vi "AlGaInPAs_Layer2.vi"(2 "Debug Mode":bool, 4 "State":enum16{"Edit", "Start", "Run", "End", "Idle"}(ring), 5 "Argument List In":string[](array[string])) -> (1 "Argument List Out":string[](array[string]))   [LabVIEW 2011]
panel:
  in  "AsH3 Flow":dbl
  in  "AsH3 run":bool
  in  "Al_run":bool
  in  "Al Flow":dbl
  in  "PH3 run":bool
  in  "In run":bool
  in  "Ga run":bool
  in  "PH3 Flow":dbl
  in  "In Flow":dbl
  in  "Ga Flow":dbl
  in  "Cancel":bool
  in  "OK":bool
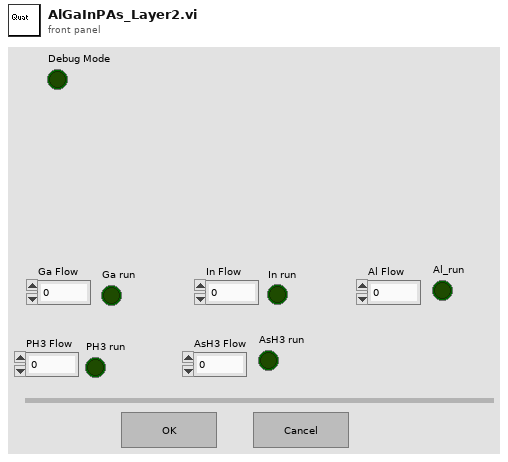
[diagram p1: front panel]
types:
  T1 = enum16{"Discrete", "Continuous", "Instantaneous"}
  T2 = enum32{"Invalid", "Default", "Floating", "Floating/Auto-Hide", "Modal"}
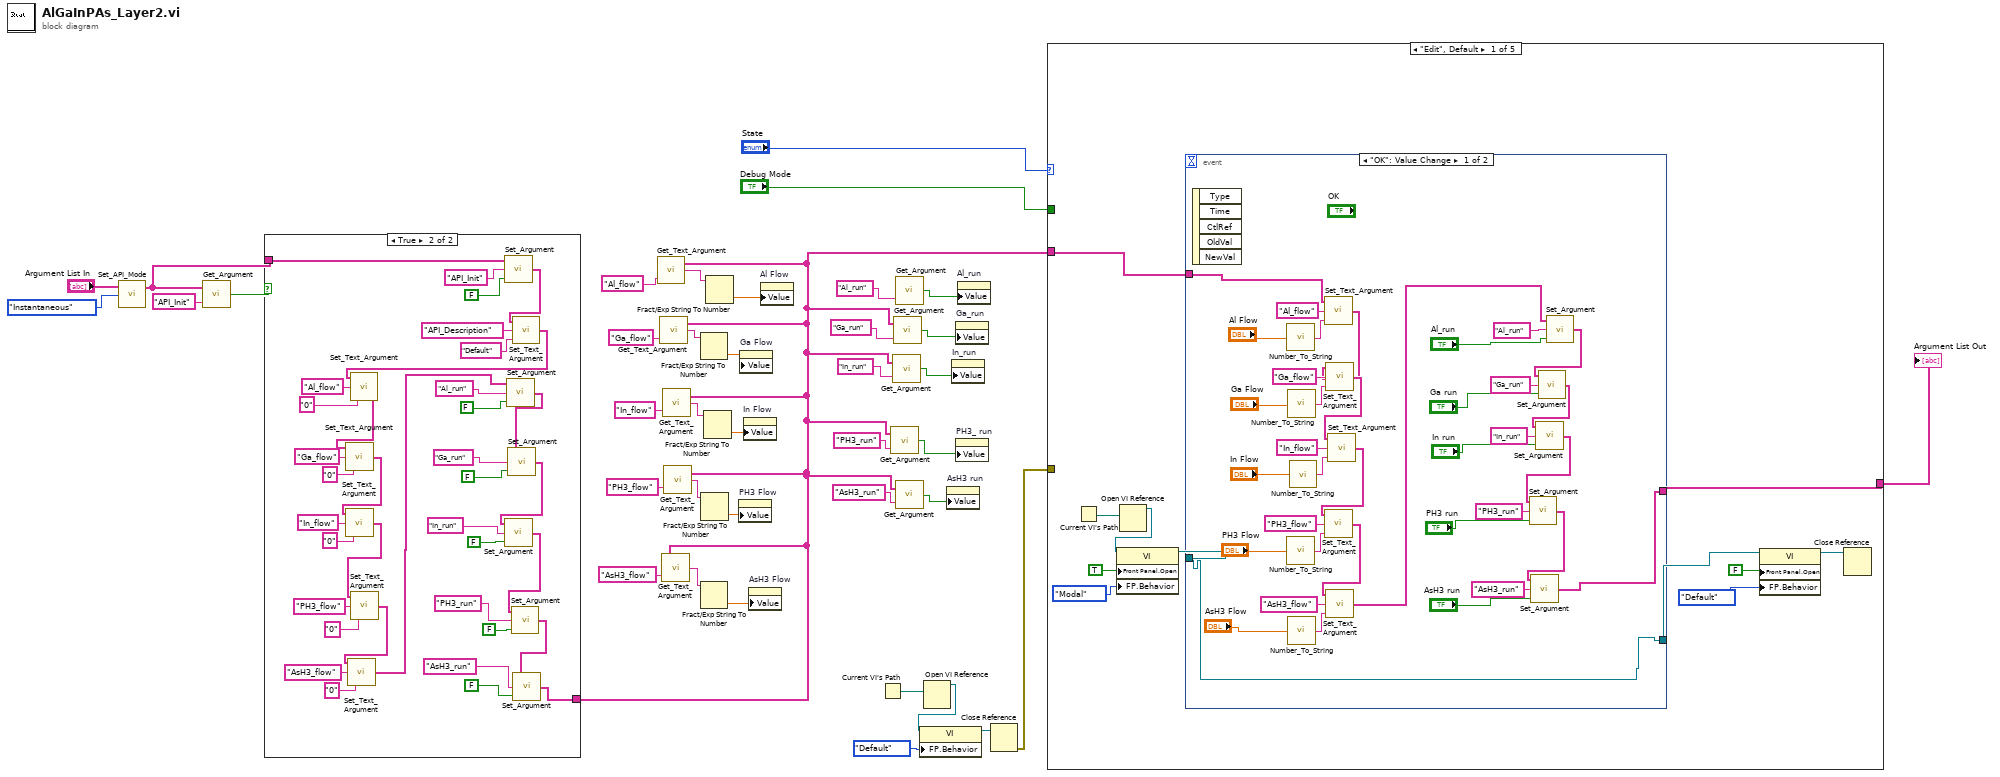
[diagram p0: block diagram]
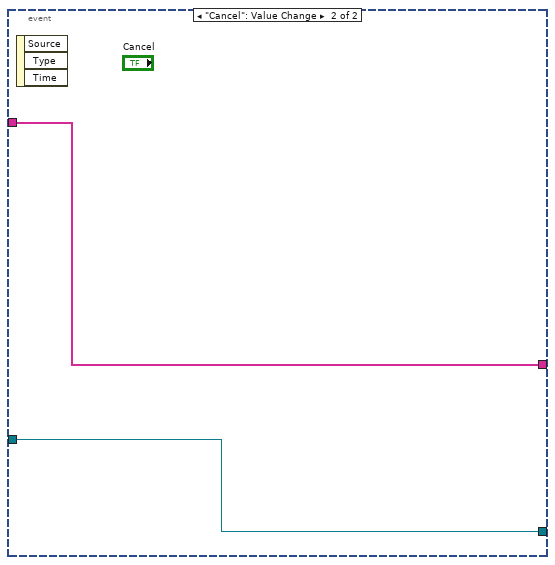
[diagram p3: hidden frame]
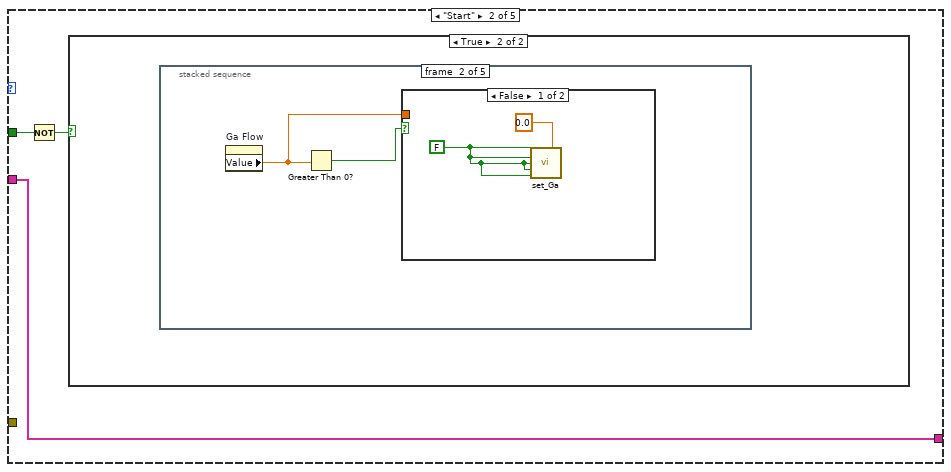
[diagram p4: hidden frame]
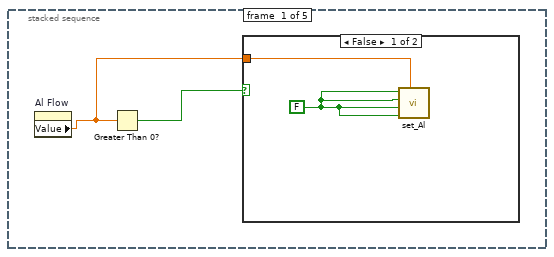
[diagram p6: hidden frame]
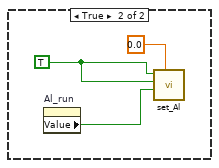
[diagram p7: hidden frame]
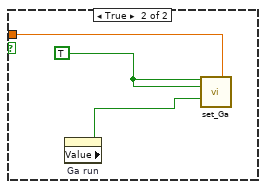
[diagram p8: hidden frame]
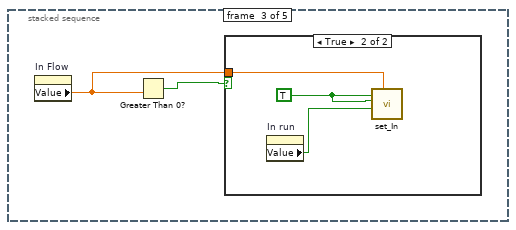
[diagram p9: hidden frame]
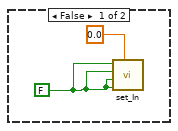
[diagram p10: hidden frame]
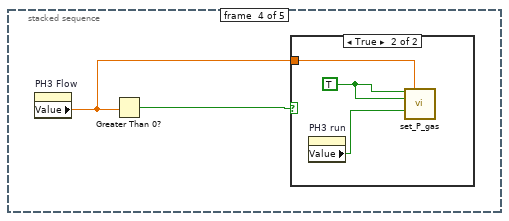
[diagram p11: hidden frame]
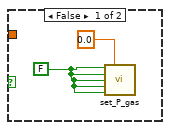
[diagram p12: hidden frame]
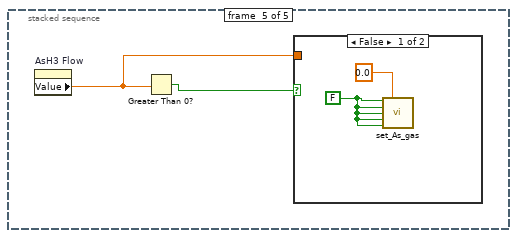
[diagram p13: hidden frame]
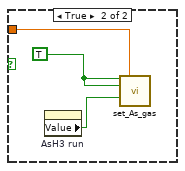
[diagram p14: hidden frame]
diagram:
  n1 = call "Set_API_Mode.vi"("API Mode"=T1."Instantaneous", "Argument List In"="Argument List In") -> ("Argument List Out"=w26:string[])  [unwired: 2 out]
  n2 = call "Get_Argument.vi"("Argument"="API_Init", "Argument List"=w26) -> ("Enabled"=w27:bool)
  n3 = case shown="True" w27 {
    tunnel: w26 -> [w40 w77]
    tunnel: [w40 w53] -> w5
    frame False {
    }
    frame True {
      n4 = call "Set_Argument.vi"("Enable"=FALSE, "Argument"="API_Init", "Argument List In"=w77) -> ("Argument List Out"=w74:string[])
      n5 = call "Set_Text_Argument.vi"("Text"="Default", "Argument"="API_Description", "Argument List In"=w74) -> ("Argument List Out"=w45:string[])
      n6 = call "Set_Text_Argument.vi"("Text"="0", "Argument"="Al_flow", "Argument List In"=w45) -> ("Argument List Out"=w44:string[])
      n7 = call "Set_Text_Argument.vi"("Text"="0", "Argument"="Ga_flow", "Argument List In"=w44) -> ("Argument List Out"=w67:string[])
      n8 = call "Set_Text_Argument.vi"("Text"="0", "Argument"="In_flow", "Argument List In"=w67) -> ("Argument List Out"=w43:string[])
      n9 = call "Set_Text_Argument.vi"("Text"="0", "Argument"="PH3_flow", "Argument List In"=w43) -> ("Argument List Out"=w55:string[])
      n10 = call "Set_Text_Argument.vi"("Text"="0", "Argument"="AsH3_flow", "Argument List In"=w55) -> ("Argument List Out"=w42:string[])
      n11 = call "Set_Argument.vi"("Enable"=FALSE, "Argument"="Al_run", "Argument List In"=w42) -> ("Argument List Out"=w48:string[])
      n12 = call "Set_Argument.vi"("Enable"=FALSE, "Argument"="Ga_run", "Argument List In"=w48) -> ("Argument List Out"=w58:string[])
      n13 = call "Set_Argument.vi"("Enable"=FALSE, "Argument"="In_run", "Argument List In"=w58) -> ("Argument List Out"=w41:string[])
      n14 = call "Set_Argument.vi"("Enable"=FALSE, "Argument"="PH3_run", "Argument List In"=w41) -> ("Argument List Out"=w51:string[])
      n15 = call "Set_Argument.vi"("Enable"=FALSE, "Argument"="AsH3_run", "Argument List In"=w51) -> ("Argument List Out"=w53:string[])
    }
  }
  n16 = call "Get_Text_Argument.vi"("Argument"="Al_flow", "Argument List"=w5) -> ("Text"=w6:string)
  n17 = call "Get_Text_Argument.vi"("Argument"="Ga_flow", "Argument List"=w5) -> ("Text"=w22:string)
  n18 = call "Get_Text_Argument.vi"("Argument"="AsH3_flow", "Argument List"=w5) -> ("Text"=w18:string)
  n19 = call "Get_Text_Argument.vi"("Argument"="In_flow", "Argument List"=w5) -> ("Text"=w20:string)
  n20 = call "Get_Text_Argument.vi"("Argument"="PH3_flow", "Argument List"=w5) -> ("Text"=w17:string)
  n21 = Fract/Exp String To Number(string=w22) -> (number=w21:dbl)  [unwired: 4 out]
  n22 = Fract/Exp String To Number(string=w18) -> (number=w1:dbl)  [unwired: 4 out]
  n23 = Fract/Exp String To Number(string=w17) -> (number=w16:dbl)  [unwired: 4 out]
  n24 = Fract/Exp String To Number(string=w20) -> (number=w19:dbl)  [unwired: 4 out]
  n25 = Fract/Exp String To Number(string=w6) -> (number=w2:dbl)  [unwired: 4 out]
  n26 = property on="PH3 Flow" class="DigNum (strict)"("Value"=w16) -> ()  [unwired: 2 in, 2 out]
  n27 = property on="Ga Flow" class="DigNum (strict)"("Value"=w21) -> ()  [unwired: 2 in, 2 out]
  n28 = property on="In Flow" class="DigNum (strict)"("Value"=w19) -> ()  [unwired: 2 in, 2 out]
  n29 = property on="AsH3 Flow" class="DigNum (strict)"("Value"=w1) -> ()  [unwired: 2 in, 2 out]
  n30 = property on="Al Flow" class="DigNum (strict)"("Value"=w2) -> ()  [unwired: 2 in, 2 out]
  n31 = Current VI's Path() -> (path=w35:path)
  n32 = call "Get_Argument.vi"("Argument"="PH3_run", "Argument List"=w5) -> ("Enabled"=w12:bool)
  n33 = call "Get_Argument.vi"("Argument"="In_run", "Argument List"=w5) -> ("Enabled"=w13:bool)
  n34 = call "Get_Argument.vi"("Argument"="Ga_run", "Argument List"=w5) -> ("Enabled"=w14:bool)
  n35 = call "Get_Argument.vi"("Argument"="Al_run") -> ("Enabled"=w4:bool)  [unwired: 1 in]
  n36 = call "Get_Argument.vi"("Argument"="AsH3_run", "Argument List"=w5) -> ("Enabled"=w3:bool)
  n37 = Open VI Reference(vi path=w35) -> (vi reference=w34:refnum<vi>)  [unwired: 1 in, 5 out]
  n38 = property class="VI"(reference=w34, "FP.Behavior"=T2."Default" ("Front Panel Window:Behavior")) -> (reference out=w32:refnum<vi>)  [unwired: 1 in, 1 out]
  n39 = property on="AsH3 run" class="Bool (strict)"("Value"=w3) -> ()  [unwired: 2 in, 2 out]
  n40 = property on="In_run" class="Bool (strict)"("Value"=w13) -> ()  [unwired: 2 in, 2 out]
  n41 = property on="Ga_run" class="Bool (strict)"("Value"=w14) -> ()  [unwired: 2 in, 2 out]
  n42 = property on="PH3_ run" class="Bool (strict)"("Value"=w12) -> ()  [unwired: 2 in, 2 out]
  n43 = property on="Al_run" class="Bool (strict)"("Value"=w4) -> ()  [unwired: 2 in, 2 out]
  n44 = Close Reference(reference=w32) -> (error out=w31:errorcluster)  [unwired: 1 in]
  n45 = case shown="\"Edit\", Default" "State" {
    tunnel: [w88 w130 w166 w167 w168] -> w38
    tunnel: w5 -> [w87 w130 w166 w167 w168]
    tunnel: "Debug Mode" -> [_ w129 _ _ _]
    tunnel: w31 -> [_ _ _ _ _]
    frame "Edit", Default {
      n46 = Current VI's Path() -> (path=w82:path)
      n47 = Open VI Reference(vi path=w82) -> (vi reference=w81:refnum<vi>)  [unwired: 1 in, 5 out]
      n48 = property class="VI"(reference=w81, "Front Panel.Open"=TRUE ("Front Panel Window:Open"), "FP.Behavior"=T2."Modal" ("Front Panel Window:Behavior")) -> (reference out=w85:refnum<vi>)  [unwired: 1 in, 1 out]
      n49 = event shown="[0] \"OK\": Value Change" {
        selector: _ -> [_ _]
        dyn-events: _ -> [_ _]
        timeout: _ -> [_ _]
        tunnel: w87 -> [w98 w126]
        tunnel: [w105 w126] -> w88
        tunnel: [w89 w127] -> w84
        tunnel: w85 -> [w89 w127]
        event "OK": Value Change {
          n50 = event-data() -> ()  [unwired: 6 out]
          n51 = call "Number_To_String.vi"("Number"="Al Flow") -> ("String"=w99:string)
          n52 = call "Number_To_String.vi"("Number"="PH3 Flow") -> ("String"=w117:string)
          n53 = call "Number_To_String.vi"("Number"="Ga Flow") -> ("String"=w124:string)
          n54 = call "Number_To_String.vi"("Number"="AsH3 Flow") -> ("String"=w95:string)
          n55 = call "Number_To_String.vi"("Number"="In Flow") -> ("String"=w121:string)
          n56 = call "Set_Text_Argument.vi"("Text"=w99, "Argument"="Al_flow", "Argument List In"=w98) -> ("Argument List Out"=w97:string[])
          n57 = call "Set_Text_Argument.vi"("Text"=w124, "Argument"="Ga_flow", "Argument List In"=w97) -> ("Argument List Out"=w120:string[])
          n58 = call "Set_Text_Argument.vi"("Text"=w121, "Argument"="In_flow", "Argument List In"=w120) -> ("Argument List Out"=w92:string[])
          n59 = call "Set_Text_Argument.vi"("Text"=w117, "Argument"="PH3_flow", "Argument List In"=w92) -> ("Argument List Out"=w93:string[])
          n60 = call "Set_Text_Argument.vi"("Text"=w95, "Argument"="AsH3_flow", "Argument List In"=w93) -> ("Argument List Out"=w94:string[])
          n61 = call "Set_Argument.vi"("Enable"="Al_run", "Argument"="Al_run", "Argument List In"=w94) -> ("Argument List Out"=w91:string[])
          n62 = call "Set_Argument.vi"("Enable"="Ga run", "Argument"="Ga_run", "Argument List In"=w91) -> ("Argument List Out"=w109:string[])
          n63 = call "Set_Argument.vi"("Enable"="In run", "Argument"="In_run", "Argument List In"=w109) -> ("Argument List Out"=w103:string[])
          n64 = call "Set_Argument.vi"("Enable"="PH3 run", "Argument"="PH3_run", "Argument List In"=w103) -> ("Argument List Out"=w104:string[])
          n65 = call "Set_Argument.vi"("Enable"="AsH3 run", "Argument"="AsH3_run", "Argument List In"=w104) -> ("Argument List Out"=w105:string[])
        }
        event "Cancel": Value Change {
          n66 = event-data() -> ()  [unwired: 4 out]
        }
      }
      n67 = property class="VI"(reference=w84, "Front Panel.Open"=FALSE ("Front Panel Window:Open"), "FP.Behavior"=T2."Default" ("Front Panel Window:Behavior")) -> (reference out=w78:refnum<vi>)  [unwired: 1 in, 1 out]
      n68 = Close Reference(reference=w78) -> ()  [unwired: 1 in, 1 out]
    }
    frame "Start" {
      n69 = Not(x=w129) -> (.not. x?=w128:bool)
      n70 = case shown="True" w128 {
        frame False {
        }
        frame True {
          n71 = stacked-sequence {
            frame #0 {
              n72 = property on="Al Flow" class="DigNum (strict)"() -> ("Value"=w131:dbl)  [unwired: 2 in, 2 out]
              n73 = Greater Than 0?(x=w131) -> (x > 0?=w132:bool)
              n74 = case shown="False" w132 {
                tunnel: w131 -> [w134 _]
                frame False {
                  w133 = FALSE ("Al Active")
                  n75 = call "set_Al.vi"("Aluminum Flow"=w134, "Al Remote"=w133, "Al Run"=w133, "Al Bubbler"=w133, "Al Active"=w133) -> ()  [unwired: 5 out]
                }
                frame True {
                  w135 = TRUE ("Al Active")
                  n76 = property on="Al_run" class="Bool (strict)"() -> ("Value"=w137:bool)  [unwired: 2 in, 2 out]
                  n77 = call "set_Al.vi"("Aluminum Flow"=0.0, "Al Run"=w137, "Al Bubbler"=w135, "Al Active"=w135) -> ()  [unwired: 1 in, 5 out]
                }
              }
            }
            frame #1 {
              n78 = property on="Ga Flow" class="DigNum (strict)"() -> ("Value"=w138:dbl)  [unwired: 2 in, 2 out]
              n79 = Greater Than 0?(x=w138) -> (x > 0?=w139:bool)
              n80 = case shown="False" w139 {
                tunnel: w138 -> [_ w143]
                frame False {
                  w140 = FALSE ("Ga Active")
                  n81 = call "set_Ga.vi"("Ga Active"=w140, "Ga Flow 1"=0.0, "Ga Bubbler"=w140, "Ga H2 Dilute"=w140, "Ga Run"=w140, "Ga Remote"=w140) -> ()  [unwired: 2 in, 8 out]
                }
                frame True {
                  w142 = TRUE ("Ga Active")
                  n82 = property on="Ga run" class="Bool (strict)"() -> ("Value"=w144:bool)  [unwired: 2 in, 2 out]
                  n83 = call "set_Ga.vi"("Ga Active"=w142, "Ga Flow 1"=w143, "Ga Bubbler"=w142, "Ga Run"=w144) -> ()  [unwired: 4 in, 8 out]
                }
              }
            }
            frame #2 {
              n84 = property on="In Flow" class="DigNum (strict)"() -> ("Value"=w145:dbl)  [unwired: 2 in, 2 out]
              n85 = Greater Than 0?(x=w145) -> (x > 0?=w146:bool)
              n86 = case shown="True" w146 {
                tunnel: w145 -> [_ w151]
                frame False {
                  w148 = FALSE ("In Remote")
                  n87 = call "set_In.vi"("Indium Flow"=0.0, "In Remote"=w148, "In Run"=w148, "In Bubbler"=w148, "In Active"=w148) -> ()  [unwired: 5 out]
                }
                frame True {
                  w150 = TRUE ("In Run")
                  n88 = property on="In run" class="Bool (strict)"() -> ("Value"=w149:bool)  [unwired: 2 in, 2 out]
                  n89 = call "set_In.vi"("Indium Flow"=w151, "In Run"=w149, "In Bubbler"=w150, "In Active"=w150) -> ()  [unwired: 1 in, 5 out]
                }
              }
            }
            frame #3 {
              n90 = property on="PH3 Flow" class="DigNum (strict)"() -> ("Value"=w152:dbl)  [unwired: 2 in, 2 out]
              n91 = Greater Than 0?(x=w152) -> (x > 0?=w153:bool)
              n92 = case shown="True" w153 {
                tunnel: w152 -> [_ w158]
                frame False {
                  w154 = FALSE ("P_Gas Active")
                  n93 = call "set_P_gas.vi"("P_Gas Active"=w154, "P_Gas Flow"=0.0, "P_Gas In"=w154, "P_Gas H2 In"=w154, "P_Gas Run"=w154, "P_Gas Remote"=w154) -> ()  [unwired: 10 out]
                }
                frame True {
                  w156 = TRUE ("P_Gas Active")
                  n94 = property on="PH3 run" class="Bool (strict)"() -> ("Value"=w157:bool)  [unwired: 2 in, 2 out]
                  n95 = call "set_P_gas.vi"("P_Gas Active"=w156, "P_Gas Flow"=w158, "P_Gas In"=w156, "P_Gas Run"=w157) -> ()  [unwired: 2 in, 10 out]
                }
              }
            }
            frame #4 {
              n96 = property on="AsH3 Flow" class="DigNum (strict)"() -> ("Value"=w160:dbl)  [unwired: 2 in, 2 out]
              n97 = Greater Than 0?(x=w160) -> (x > 0?=w159:bool)
              n98 = case shown="False" w159 {
                tunnel: w160 -> [_ w165]
                frame False {
                  w161 = FALSE ("As_Gas Active")
                  n99 = call "set_As_gas.vi"("As_Gas Active"=w161, "As_Gas Flow"=0.0, "As_Gas In"=w161, "As_Gas H2"=w161, "As_Gas Run"=w161, "As_Gas Remote"=w161) -> ()  [unwired: 10 out]
                }
                frame True {
                  w163 = TRUE ("As_Gas Active")
                  n100 = property on="AsH3 run" class="Bool (strict)"() -> ("Value"=w164:bool)  [unwired: 2 in, 2 out]
                  n101 = call "set_As_gas.vi"("As_Gas Active"=w163, "As_Gas Flow"=w165, "As_Gas In"=w163, "As_Gas Run"=w164) -> ()  [unwired: 2 in, 10 out]
                }
              }
            }
          }
        }
      }
    }
    frame "Run" {
    }
    frame "End" {
    }
    frame "Idle" {
    }
  }
  "Argument List Out" <- w38
